vi "jsonInsertU64.vi"(8 "error in (no error)":errorcluster, 9 "value":u64, 10 "path":string, 11 "d in":i64) -> (0 "error out":errorcluster, 1 "replaced?":bool, 3 "d out":i64)   [LabVIEW 2015, in "rapidjson wrapper.lvlib"]
uses:
  rapidjson wrapper.lvlib
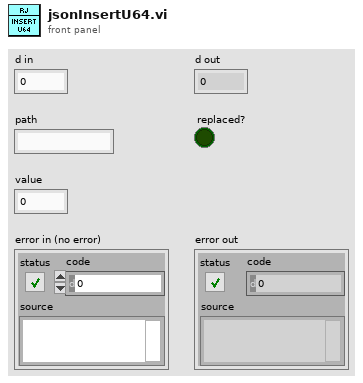
[diagram p1: front panel]
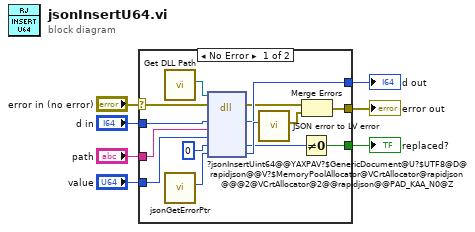
[diagram p0: block diagram]
diagram:
  n1 = case shown="No Error" "error in (no error)" {
    selector: "error in (no error)" -> [w14 w23]
    tunnel: [w11 w23] -> w7
    tunnel: "value" -> [w18 _]
    tunnel: "d in" -> [w17 w22]
    tunnel: "path" -> [w16 _]
    tunnel: [w15 w22] -> w2
    tunnel: [w9 _] -> w1
    frame No Error {
      n2 = call "Get DLL Path.vi"() -> ("Path"=w21:path)  [unwired: 11 in]
      n3 = call "jsonGetErrorPtr.vi"() -> ("return type"=w19:i64)  [unwired: 10 in, 1 out]
      n4 = dll-call lib="C:/Users/tblair/Documents/Git Projects/rapidjson-for-LabVIEW/lvrjs/Debug/lvrjs.dll" fn="?jsonInsertUint64@@YAXPAV?$GenericDocument@U?$UTF8@D@rapidjson@@V?$MemoryPoolAllocator@VCrtAllocator@rapidjson@@@2@VCrtAllocator@2@@rapidjson@@PAD_KAA_N0@Z"(path in=w21, error in=w14, "d"=w17, "path"=w16, "value"=w18, "replaced"=0, "jsonError"=w19) -> (error out=w13:errorcluster, "d"=w15:i64, "replaced"=w10:i32, "jsonError"=w20:i64)  [unwired: 4 in, 1 out]
      n5 = call "JSON error to LV error.vi"("jsonError"=w20) -> ("error out"=w12:errorcluster)  [unwired: 10 in]
      n6 = Not Equal To 0?(x=w10) -> (x != 0?=w9:bool)
      n7 = Merge Errors(w13, w12) -> (w11:errorcluster)
    }
    frame Error {
    }
  }
  "error out" <- w7
  "d out" <- w2
  "replaced?" <- w1
